vi "Fit Font Size to Box.vi"(8 "text":string, 9 "box rect":T2, 10 "box center":cluster{"x":i16, "y":i16}, 11 "font name":string="Helvetica") -> (3 "font":T1)   [LabVIEW 2017, in "NI_Robotics_Control Utilities.lvlib"]
uses:
  <vilib>/robotics/Controls/Utilities/NI_Robotics_Control Utilities.lvlib
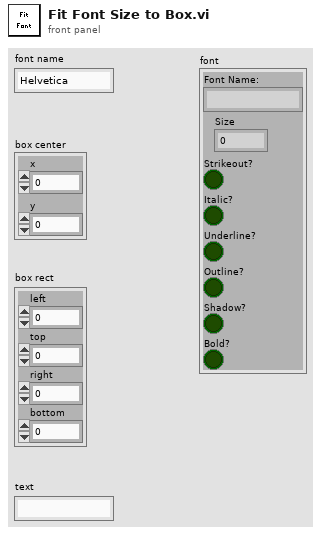
[diagram p1: front panel]
types:
  T1 = cluster{"Font Name:":string, "Size":i16, "Strikeout?":bool, "Italic?":bool, "Underline?":bool, "Outline?":bool, "Shadow?":bool, "Bold?":bool}
  T2 = cluster{"left":i16, "top":i16, "right":i16, "bottom":i16}
  T3 = enum16{"User-specified Font", "Application Font", "System Font", "Dialog Font"}
  T4 = cluster{"horizontal":enum16{"left", "center", "right"}, "vertical":enum16{"top", "center", "bottom"}}
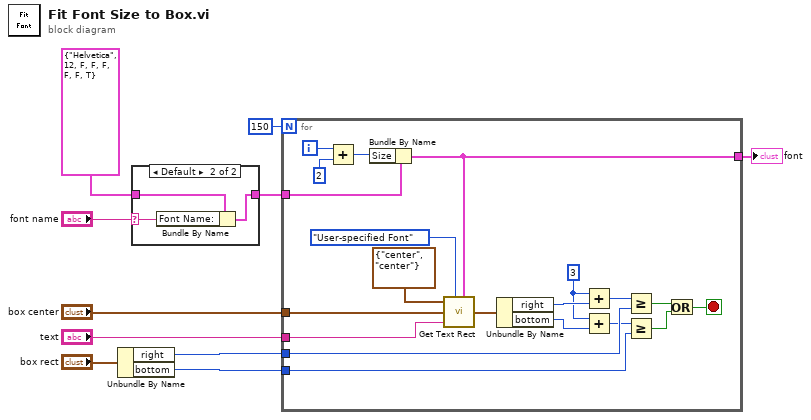
[diagram p0: block diagram]
diagram:
  n1 = Unbundle By Name("box rect") -> ("right"=w5:i16, "bottom"=w4:i16)
  n2 = case shown="Default" "font name" {
    selector: "font name" -> [_ w12]
    tunnel: T1 {"Font Name:"="Helvetica", "Size"=12, "Strikeout?"=FALSE, "Italic?"=FALSE, "Underline?"=FALSE, "Outline?"=FALSE, "Shadow?"=FALSE, "Bold?"=TRUE} ("[user-specified font]") -> [w11 w14]
    tunnel: [w11 w13] -> w7
    frame "" {
    }
    frame Default {
      n3 = Bundle By Name(cluster=w14, "Font Name:"=w12) -> (w13:T1)
    }
  }
  n4 = for {
    N: 150 -> [_]
    tunnel: "box center" -> [w34]
    tunnel: w7 -> [w26]
    tunnel: w5 -> [w20]
    tunnel: w4 -> [w18]
    tunnel: "text" -> [w30]
    tunnel: [w25] -> w2
    i -> [w29]
    stop <- w15 stop-if-true
    w22 = i16 3 ("x")
    n5 = Add(x=w29, y=2) -> (x+y=w27:i32)
    n6 = Bundle By Name(cluster=w26, "Size"=w27) -> (w25:T1)
    n7 = call <vilib>:"Get Text Rect.vi"("alignment(left, top)"=T4 {"horizontal"=enum."center", "vertical"=enum."center"}, "desired font(Application)"=T3."User-specified Font", "origin(0,0)"=w34, "text"=w30, "[user-specified font]"=w25) -> ("rect"=w31:T2)  [unwired: 4 in]
    n8 = Unbundle By Name(w31) -> ("right"=w24:i16, "bottom"=w23:i16)
    n9 = Add(x=w22, y=w24) -> (x+y=w21:i16)
    n10 = Add(x=w22, y=w23) -> (x+y=w19:i16)
    n11 = Greater Or Equal?(x=w21, y=w20) -> (x >= y?=w17:bool)
    n12 = Greater Or Equal?(x=w19, y=w18) -> (x >= y?=w16:bool)
    n13 = Or(x=w17, y=w16) -> (x .or. y?=w15:bool)
  }
  "font" <- w2
